vi "GlobalVariableChanger.vi"(8 "DataFlowIn":bool) -> (0 "DataFlowOut":bool)   [LabVIEW 2016]
uses:
  LabVIEW Data/Zeus Dashboard/VisionProcessingBoolean.vi
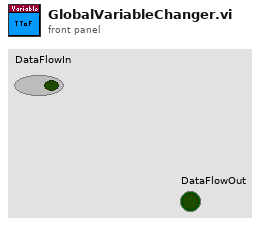
[diagram p1: front panel]
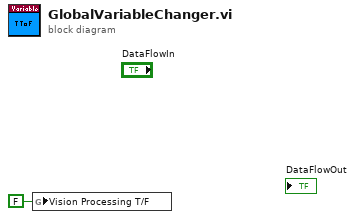
[diagram p0: block diagram]
diagram:
  n1 = global write "VisionProcessingBoolean.vi" "Vision Processing T/F"(FALSE ("Vision Processing T/F")) -> ()
